vi "Initialize Language.vi"(8 "error in (no error)":errorcluster) -> (0 "error out":errorcluster)   [LabVIEW 2019, in "FootScan Engine.lvlib"]
uses:
  FootScan Engine.lvlib
panel:
  # "Input"
  # "Output"
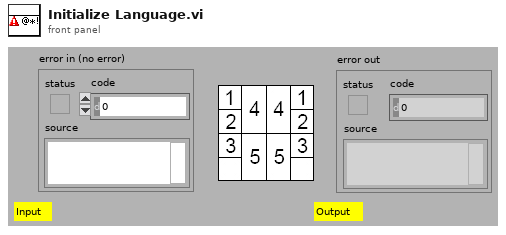
[diagram p1: front panel]
types:
  T1 = typedef "FootScan Engine.lvlib/Interface Refnums.ctl" = cluster{"Button 0 Refnum":refnum<vi>, "Exit Refnum":refnum<vi>}
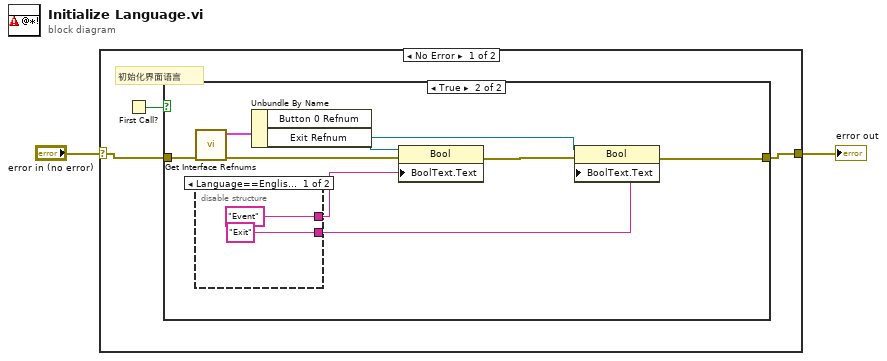
[diagram p0: block diagram]
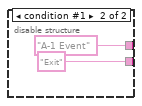
[diagram p3: hidden frame]
diagram:
  n1 = case shown="No Error" "error in (no error)" {
    selector: "error in (no error)" -> [w4 w20]
    tunnel: [w3 w20] -> w1
    frame No Error {
      # "初始化界面语言"
      n2 = First Call?() -> (First Call?: T/F=w5:bool)
      n3 = case shown="True" w5 {
        tunnel: w4 -> [w6 w14]
        tunnel: [w6 w11] -> w3
        frame False {
        }
        frame True {
          n4 = call "Get Interface Refnums.vi"("error in (no error)"=w14) -> ("error out"=w15:errorcluster, "Button 0 Refnum Out"=w10:T1)  [unwired: 9 in]
          n5 = disable-structure shown="Language==English, default" {
            disable-tunnel: ["Event" ("Boolean Text.Text") "A-1 Event" ("Boolean Text.Text")] -> w13
            disable-tunnel: ["Exit" ("Boolean Text.Text") "Exit" ("Boolean Text.Text")] -> w12
            frame condition #0 (active) {
            }
            frame condition #1 {
            }
          }
          n6 = Unbundle By Name(w10) -> ("Button 0 Refnum"=w9:refnum<vi>, "Exit Refnum"=w7:refnum<vi>)
          n7 = property class="Bool"(reference=w9, error in=w15, "BoolText.Text"=w13) -> (error out=w8:errorcluster)  [unwired: 1 out]
          n8 = property class="Bool"(reference=w7, error in=w8, "BoolText.Text"=w12) -> (error out=w11:errorcluster)  [unwired: 1 out]
        }
      }
    }
    frame Error {
    }
  }
  "error out" <- w1
